vi "save tiff.vi"(8 "error in (no error)":errorcluster, 11 "Cascade in":refnum<class "Cascade.lvclass">) -> (0 "error out":errorcluster, 3 "Cascade out":refnum<class "Cascade.lvclass">)   [LabVIEW 2012, in "Cascade.lvclass"]
uses:
  Cascade.lvclass
  Cascade.lvclass/Cascade.ctl
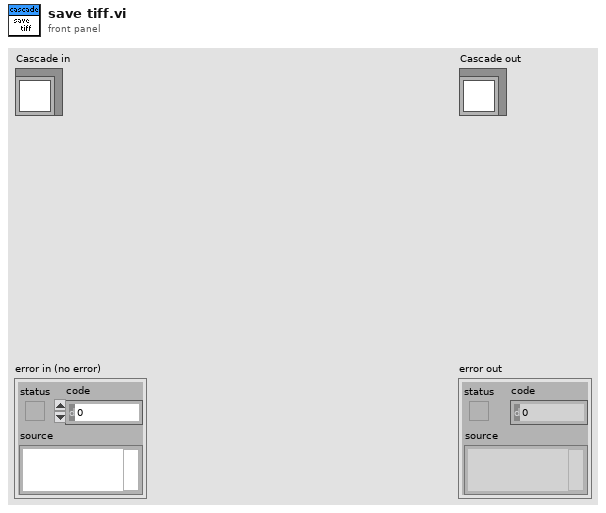
[diagram p1: front panel]
types:
  T1 = typedef "IMAQ Image.ctl" = refnum<image>
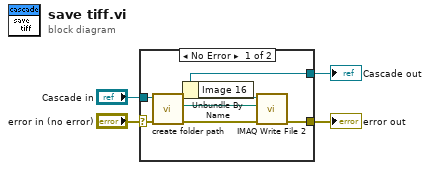
[diagram p0: block diagram]
diagram:
  n1 = case shown="No Error" "error in (no error)" {
    selector: "error in (no error)" -> [w9 w13]
    tunnel: [w10 w13] -> w3
    tunnel: [w5 w12] -> w1
    tunnel: "Cascade in" -> [w6 w12]
    frame No Error {
      n2 = call-dynamic "create folder path.vi"("error in (no error)"=w9, "Cascade in"=w6) -> ("error out"=w8:errorcluster, "dup path"=w7:path, "Cascade out"=w5:refnum<class "Cascade.lvclass">)  [unwired: 7 in]
      n3 = Unbundle By Name(w5) -> ("Image 16"=w11:T1)
      n4 = call-poly "IMAQ Write File 2"("error in (no error)"=w8, "File Path"=w7, "Image"=w11) -> ("error out"=w10:errorcluster)  [unwired: 7 in, 1 out]
    }
    frame Error {
    }
  }
  "error out" <- w3
  "Cascade out" <- w1
